vi "IsEnabled.vi"(8 "error in (no error)":errorcluster, 11 "Controlador in":refnum<class "Controlador.lvclass">) -> (0 "error out":errorcluster, 2 "Boolean":bool, 3 "Controlador out":refnum<class "Controlador.lvclass">)   [LabVIEW 2018, in "Controlador.lvclass"]
uses:
  Controlador.lvclass
  Controlador.lvclass/Controlador.ctl
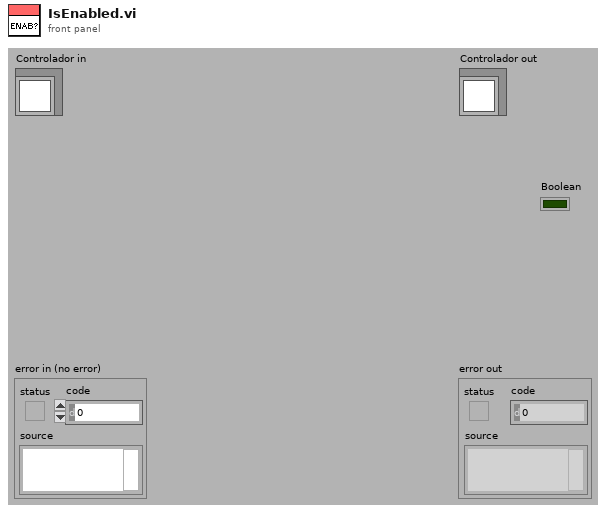
[diagram p1: front panel]
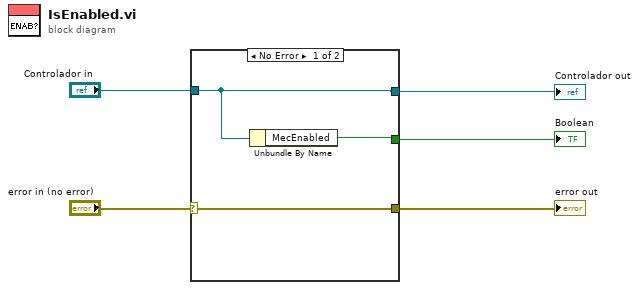
[diagram p0: block diagram]
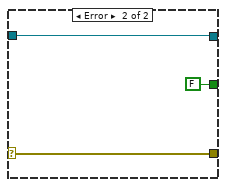
[diagram p2: hidden frame]
diagram:
  n1 = case shown="No Error" "error in (no error)" {
    selector: "error in (no error)" -> [w6 w9]
    tunnel: "Controlador in" -> [w8 w10]
    tunnel: [w6 w9] -> w2
    tunnel: [w8 w10] -> w4
    tunnel: [w7 FALSE ("MecEnabled")] -> w3
    frame No Error {
      n2 = Unbundle By Name(w8) -> ("MecEnabled"=w7:bool)
    }
    frame Error {
    }
  }
  "error out" <- w2
  "Controlador out" <- w4
  "Boolean" <- w3
